vi "Initiate_Motion.vi"(6 "Error In":errorcluster, 8 "Node":i32, 9 "Serial In":refnum<visa-resource-name>) -> (0 "Error Out":errorcluster, 3 "Serial Out":refnum<visa-resource-name>)   [LabVIEW 2018]
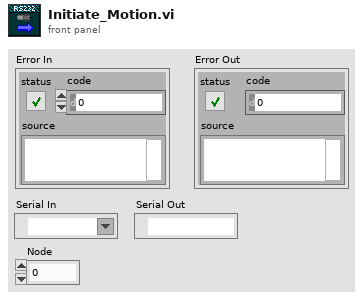
[diagram p1: front panel]
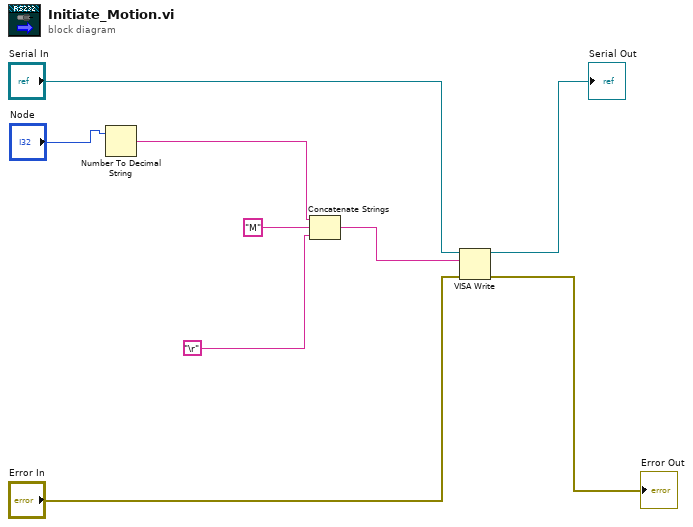
[diagram p0: block diagram]
diagram:
  n1 = Number To Decimal String(number="Node") -> (decimal integer string=w4:string)  [unwired: 1 in]
  n2 = Concatenate Strings(w4, "M" ("string"), "\r") -> (w3:string)
  n3 = VISA Write(VISA resource name="Serial In", write buffer=w3, error in (no error)="Error In") -> (VISA resource name out=→"Serial Out":refnum<visa-resource-name>, error out=→"Error Out":errorcluster)  [unwired: 1 out]
